vi "Longitudinal-Radial Distance_2011.vi"(3 "Image (Counts)":dbl[][](array[numeric]), 4 "ROI infos":T3={"npix-X"=512, "npix-Y"=384, "Left [pix]"=0.0, "Top [pix]"=0.0}, 5 "Screen&Camera":T1={"Screen Orientation"="Regular", "Screen angle"="Flat", "Lens"=enum."FL1-f8x08", "Calibration (mm/pix)"=1.0}) -> (0 "Z map":dbl[][](array[numeric]), 2 "R^2 map":dbl[][](array[numeric]))   [LabVIEW 2020]
uses:
  ScreenCam2_TypDEf.ctl
  CamAndObj_TypDEf.ctl
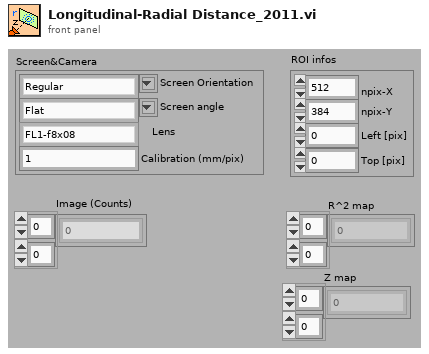
[diagram p1: front panel]
types:
  T1 = typedef "ScreenCam2_TypDEf.ctl" = cluster{"Screen Orientation":string, "Screen angle":string, "Lens":T2, "Calibration (mm/pix)":dbl}
  T2 = typedef "CamAndObj_TypDEf.ctl" = enum16{"FL1-f8x08", "FL1-f8x06", "FL1-f8", "ch300-f50", "FL2G-f8", "FL3M14-f8", "FL3M14-f8x08", "FL3M14-f8x08(2x2)", "aca720-f8", "aca1440-f8"}
  T3 = cluster{"npix-X":i32, "npix-Y":i32, "Left [pix]":dbl, "Top [pix]":dbl}
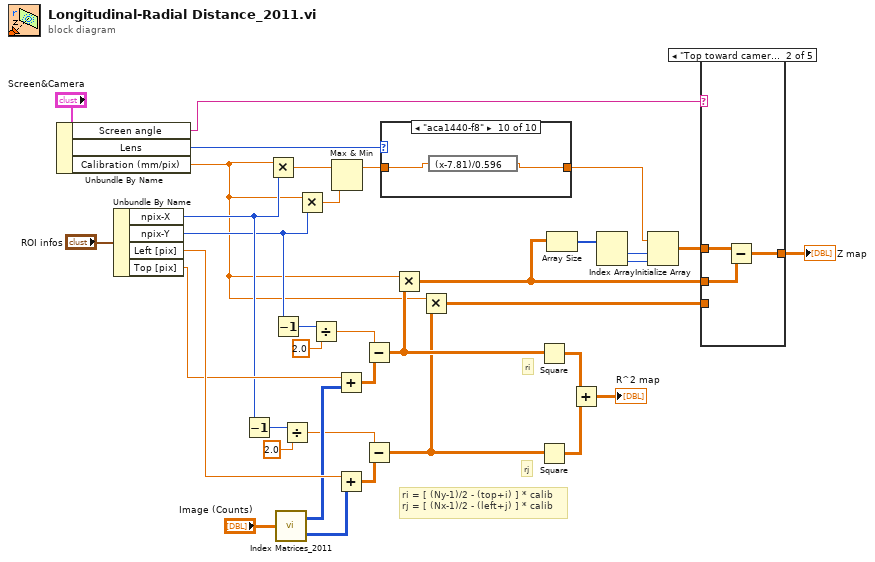
[diagram p0: block diagram]
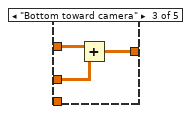
[diagram p3: hidden frame]
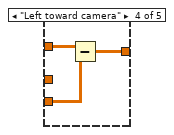
[diagram p4: hidden frame]
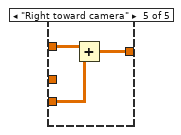
[diagram p5: hidden frame]
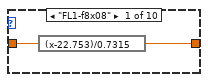
[diagram p6: hidden frame]
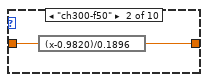
[diagram p7: hidden frame]
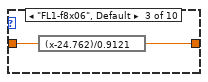
[diagram p8: hidden frame]
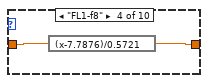
[diagram p9: hidden frame]
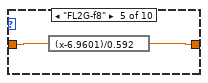
[diagram p10: hidden frame]
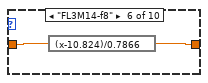
[diagram p11: hidden frame]
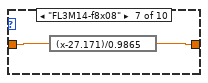
[diagram p12: hidden frame]
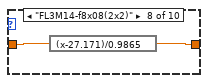
[diagram p13: hidden frame]
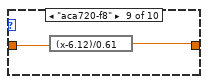
[diagram p14: hidden frame]
diagram:
  # "ri = [ (Ny-1)/2 - (top+i) ] * calib\nrj = [ (Nx-1)/2 - (left+j) ] * calib"
  # "ri"
  # "rj"
  n1 = Unbundle By Name("Screen&Camera") -> ("Screen angle"=w34:string, "Lens"=w1:T2, "Calibration (mm/pix)"=w4:dbl)
  n2 = Unbundle By Name("ROI infos") -> ("npix-X"=w21:i32, "npix-Y"=w20:i32, "Left [pix]"=w26:dbl, "Top [pix]"=w22:dbl)
  n3 = Decrement(x=w21) -> (x-1=w33:i32)
  n4 = Multiply(x=w4, y=w21) -> (x*y=w17:dbl)
  n5 = Decrement(x=w20) -> (x-1=w32:i32)
  n6 = call "Index Matrices_2011.vi"("Image In"="Image (Counts)") -> ("M(j)"=w25:i32[][], "M(i)"=w18:i32[][])  [unwired: 2 out]
  n7 = Divide(x=w33, y=2.0) -> (x/y=w13:dbl)
  n8 = Multiply(x=w4, y=w20) -> (x*y=w16:dbl)
  n9 = Divide(x=w32, y=2.0) -> (x/y=w14:dbl)
  n10 = Max & Min(x=w17, y=w16) -> (max(x,y)=w15:dbl)  [unwired: 1 out]
  n11 = Add(x=w22, y=w18) -> (x+y=w23:dbl[][])
  n12 = Add(x=w26, y=w25) -> (x+y=w24:dbl[][])
  n13 = Subtract(x=w14, y=w23) -> (x-y=w6:dbl[][])
  n14 = Subtract(x=w13, y=w24) -> (x-y=w5:dbl[][])
  n15 = case shown="\"aca1440-f8\"" w1 {
    tunnel: w15 -> [w38 w40 w42 w44 w46 w48 w50 w52 w54 w56]
    tunnel: [w37 w39 w41 w43 w45 w47 w49 w51 w53 w55] -> w9
    frame "FL1-f8x08" {
      n16 = expression code="(x-22.753)/0.7315"(w38) -> (w37:dbl)
    }
    frame "ch300-f50" {
      n17 = expression code="(x-0.9820)/0.1896"(w40) -> (w39:dbl)
    }
    frame "FL1-f8x06", Default {
      n18 = expression code="(x-24.762)/0.9121"(w42) -> (w41:dbl)
    }
    frame "FL1-f8" {
      n19 = expression code="(x-7.7876)/0.5721"(w44) -> (w43:dbl)
    }
    frame "FL2G-f8" {
      n20 = expression code="(x-6.9601)/0.592"(w46) -> (w45:dbl)
    }
    frame "FL3M14-f8" {
      n21 = expression code="(x-10.824)/0.7866"(w48) -> (w47:dbl)
    }
    frame "FL3M14-f8x08" {
      n22 = expression code="(x-27.171)/0.9865"(w50) -> (w49:dbl)
    }
    frame "FL3M14-f8x08(2x2)" {
      n23 = expression code="(x-27.171)/0.9865"(w52) -> (w51:dbl)
    }
    frame "aca720-f8" {
      n24 = expression code="(x-6.12)/0.61"(w54) -> (w53:dbl)
    }
    frame "aca1440-f8" {
      n25 = expression code="(x-7.81)/0.596"(w56) -> (w55:dbl)
    }
  }
  n26 = Multiply(x=w4, y=w6) -> (x*y=w3:dbl[][])
  n27 = Multiply(x=w4, y=w5) -> (x*y=w2:dbl[][])
  n28 = Square(x=w6) -> (x^2=w28:dbl[][])
  n29 = Square(x=w5) -> (x^2=w29:dbl[][])
  n30 = Array Size(array=w3) -> (size(s)=w10:i32[])
  n31 = Add(x=w28, y=w29) -> (x+y=→"R^2 map":dbl[][])
  n32 = Index Array(array=w10) -> (element #1=w11:i32, element #2=w12:i32)  [unwired: 2 in]
  n33 = Initialize Array(w9, w11, w12) -> (w8:dbl[][])
  n34 = case shown="\"Top toward camera\"" w34 {
    tunnel: w8 -> [w57 w60 w63 w66 w69]
    tunnel: w3 -> [_ w59 w62 _ _]
    tunnel: w2 -> [_ _ _ w65 w68]
    tunnel: [w57 w58 w61 w64 w67] -> w7
    frame "Flat", Default {
    }
    frame "Top toward camera" {
      n35 = Subtract(x=w60, y=w59) -> (x-y=w58:dbl[][])
    }
    frame "Bottom toward camera" {
      n36 = Add(x=w63, y=w62) -> (x+y=w61:dbl[][])
    }
    frame "Left toward camera" {
      n37 = Subtract(x=w66, y=w65) -> (x-y=w64:dbl[][])
    }
    frame "Right toward camera" {
      n38 = Add(x=w69, y=w68) -> (x+y=w67:dbl[][])
    }
  }
  "Z map" <- w7
